vi "242.vi"   [LabVIEW 2017]
uses:
  user.lib/_NEVSTOP/Communicable State Machine(CSM)/Communicable State Machine.lvlib
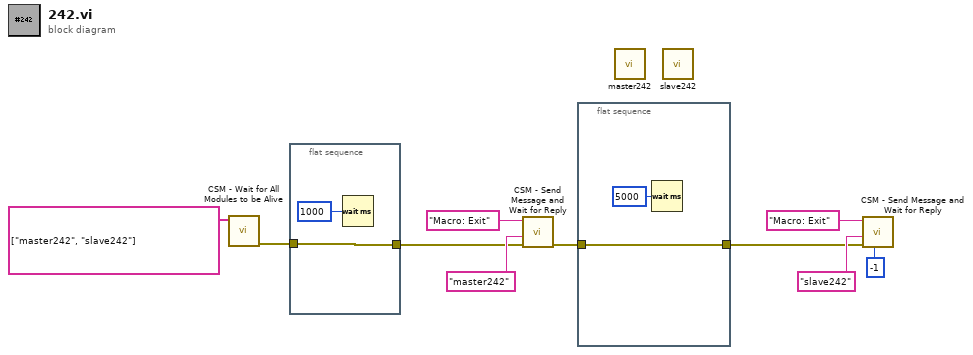
[diagram p0: block diagram]
diagram:
  n1 = call "CSM - Wait for All Modules to be Alive.vi"("CSM Names"=string[] ["master242", "slave242"] ("Module Names (in)")) -> ("error out"=w1:errorcluster)  [unwired: 8 in, 2 out]
  n2 = flat-sequence {
    tunnel: [w11] -> w2
    tunnel: w1 -> [w11]
    frame #0 {
      n3 = Wait (ms)(milliseconds to wait=u32 1000) -> ()  [unwired: 1 out]
    }
  }
  n4 = call "CSM - Send Message and Wait for Reply.vi"("Error In (No Error)"=w2, "Target Module"="master242", "State"="Macro: Exit") -> ("error out"=w4:errorcluster)  [unwired: 6 in, 2 out]
  n5 = flat-sequence {
    tunnel: [w13] -> w5
    tunnel: w4 -> [w13]
    frame #0 {
      n6 = Wait (ms)(milliseconds to wait=u32 5000) -> ()  [unwired: 1 out]
    }
  }
  n7 = call "master242.vi"() -> ()  [unwired: 12 in]
  n8 = call "slave242.vi"() -> ()  [unwired: 12 in]
  n9 = call "CSM - Send Message and Wait for Reply.vi"("Response Timeout (-2 Using Global Settings)"=-1 ("Response Timeout(5000ms)"), "Error In (No Error)"=w5, "Target Module"="slave242", "State"="Macro: Exit") -> ()  [unwired: 5 in, 3 out]
